vi "Public Key Data Authentication.vi"(4 "Public Key File":path, 6 "Private Key File":path, 7 "Address":string="localhost", 8 "Error In":errorcluster) -> (0 "Error Out":errorcluster)   [LabVIEW 2017, in "Tests.lvlib" / "Session.lvlib"]
uses:
  Session.lvlib
  Support/SSH Key Types.ctl
  <vilib>/Utility/file.llb/Is Path and Not Empty.vi
  <vilib>/Utility/sysdir.llb/Get System Directory.vi
  src/Toolkit/API/Session/Support/Public Key Memory Authentication.vi
  <vilib>/addons/_JKI Toolkits/Caraya/classes/Test/Test.lvclass
  src/Toolkit/Toolkit.lvlib
  src/Toolkit/API/Session/Session.lvclass
  <vilib>/addons/_JKI Toolkits/Caraya/classes/Assert/Assert.lvclass
  Tests.lvlib
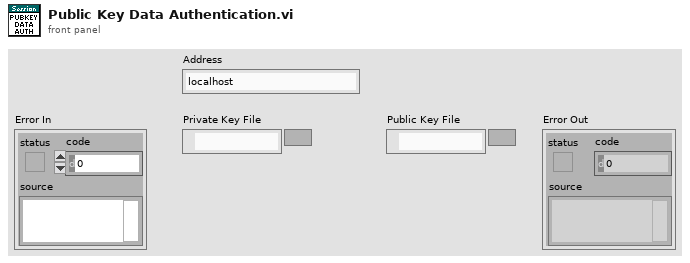
[diagram p1: front panel]
types:
  T1 = typedef "Tests.lvlib/SSH Key Types.ctl" = enum16{"Private", "Public"}
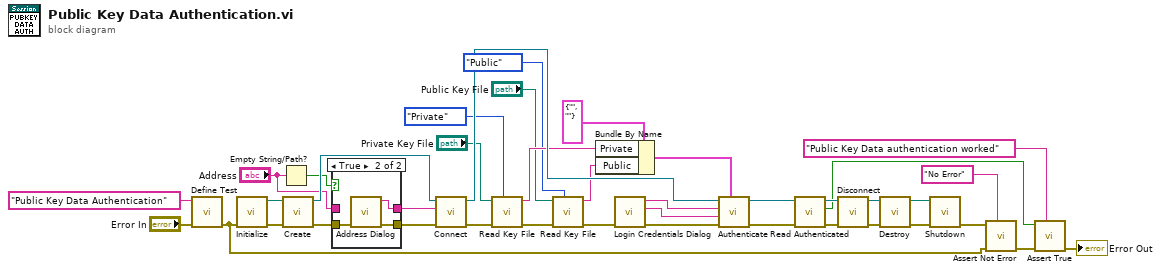
[diagram p0: block diagram]
diagram:
  n1 = call <vilib>:"Define Test.vi"("error in (no error)"="Error In", "Label (VI Title)"="Public Key Data Authentication") -> ("error out"=w32:errorcluster)  [unwired: 9 in]
  n2 = call "Initialize.vi"("Error In"=w32) -> ("Error Out"=w38:errorcluster, "lv-libssh2 Shared Library Out"=w37:path)  [unwired: 9 in]
  n3 = Empty String/Path?(string/path="Address") -> (empty?=w14:bool)
  n4 = call "Create.vi"("Error In"=w38, "lv-libssh2 Shared Library"=w37) -> ("Error Out"=w13:errorcluster, "Sesssion"=w30:refnum<class "Session.lvclass">)  [unwired: 8 in]
  n5 = case shown="True" w14 {
    tunnel: w13 -> [w41 w45]
    tunnel: [w41 w44] -> w12
    tunnel: [w42 w43] -> w11
    tunnel: "Address" -> [w42 _]
    frame False {
    }
    frame True {
      n6 = call "Address Dialog.vi"("Error In"=w45) -> ("Error Out"=w44:errorcluster, "Address Out"=w43:string)  [unwired: 9 in]
    }
  }
  n7 = call "Connect.vi"("Error In"=w12, "Address"=w11, "Session In"=w30) -> ("Error Out"=w8:errorcluster, "Sesssion Out"=w27:refnum<class "Session.lvclass">)  [unwired: 7 in]
  n8 = call "Read Key File.vi"("Key Type"=SSH_Key_Types."Private", "Error In"=w8, "Key File"="Private Key File") -> ("Error Out"=w3:errorcluster, "Key Data"=w15:string)  [unwired: 7 in]
  n9 = call "Read Key File.vi"("Key Type"=SSH_Key_Types."Public", "Error In"=w3, "Key File"="Public Key File") -> ("Error Out"=w2:errorcluster, "Key Data"=w1:string)  [unwired: 7 in]
  n10 = Bundle By Name(cluster=cluster{"Private":string, "Public":string} {"Private"="", "Public"=""} ("Keys"), "Private"=w15, "Public"=w1) -> (w16:cluster{"Private":string, "Public":string})
  n11 = call "Login Credentials Dialog.vi"("Error In"=w2) -> ("Error Out"=w9:errorcluster, "Password Out"=w18:string, "Username Out"=w19:string)  [unwired: 8 in]
  n12 = call-poly "Authenticate.vi"("Keys"=w16, "Error In"=w9, "Passphrase"=w18, "Username"=w19, "Session In"=w27) -> ("Error Out"=w25:errorcluster, "Sesssion Out"=w26:refnum<class "Session.lvclass">)  [unwired: 5 in]
  n13 = call "Read Authenticated.vi"("Error In"=w25, "Session In"=w26) -> ("Error Out"=w24:errorcluster, "Authenticated"=w21:bool, "Sesssion Out"=w23:refnum<class "Session.lvclass">)  [unwired: 7 in]
  n14 = call "Disconnect.vi"("Error In"=w24, "Session In"=w23) -> ("Error Out"=w28:errorcluster, "Sesssion Out"=w29:refnum<class "Session.lvclass">)  [unwired: 8 in]
  n15 = call "Destroy.vi"("Error In"=w28, "Session"=w29) -> ("Error Out"=w35:errorcluster, "lv-libssh2 Shared Library"=w36:path)  [unwired: 8 in]
  n16 = call "Shutdown.vi"("Error In"=w35, "lv-libssh2 Shared Library"=w36) -> ("Error Out"=w34:errorcluster)  [unwired: 9 in]
  n17 = call <vilib>:"Assert Not Error.vi"("Label"="No Error", "error in (no error)"=w32, "Not Error?"=w34) -> ("error out"=w31:errorcluster)  [unwired: 8 in]
  n18 = call <vilib>:"Assert True.vi"("Label"="Public Key Data authentication worked", "error in (no error)"=w31, "True?"=w21) -> ("error out"=→"Error Out":errorcluster)  [unwired: 8 in]
